vi "Capture System Configuration.vi"() -> ()   [LabVIEW 2024]
uses:
  <vilib>/nisyscfg/nisyscfg.lvlib
  <resource>/objmgr/nisysapi.rc
  <vilib>/Plug-In SDKs/Clients/Metadata Store V1/Metadata Store Client.lvlibp
  <vilib>/Plug-In SDKs/Clients/Metadata/Hardware Item.ctl
  <vilib>/Plug-In SDKs/Clients/Metadata/NI Metadata Types.lvlib
  <vilib>/Plug-In SDKs/Clients/Metadata/Software Item.ctl
  <vilib>/Plug-In SDKs/Clients/Metadata/Test Station.ctl
  <vilib>/Plug-In SDKs/Clients/Data Store V1/Data Store Client.lvlibp
  <vilib>/Plug-In SDKs/Clients/Metadata/Outcome.ctl
  <vilib>/Plug-In SDKs/Clients/Data Store V1/Data Store Client.lvlibp/API/Data Store V1/Test Result.ctl
  <vilib>/Plug-In SDKs/Clients/Metadata/Operator.ctl
  State Data.ctl
  <vilib>/Plug-In SDKs/Clients/Metadata/Step.ctl
  <vilib>/measure/NI_MABase.lvlib
  <vilib>/Plug-In SDKs/Clients/Metadata/Error Information.ctl
  <vilib>/Plug-In SDKs/Clients/Metadata/Extension Value.ctl
  <vilib>/Plug-In SDKs/Clients/Data Store V1/Data Store Client.lvlibp/API/Data Store V1/Publish Measurement (DBL Analog Waveform).vi
  <vilib>/Plug-In SDKs/Clients/Metadata Store V1/Metadata Store Client.lvlibp/API/Metadata Store V1/Create Hardware Item.vi
  <vilib>/Plug-In SDKs/Clients/Metadata Store V1/Metadata Store Client.lvlibp/API/Metadata Store V1/Create Software Item.vi
  <vilib>/nisyscfg/Get Installed Components.vi
  <vilib>/Plug-In SDKs/Clients/Metadata Store V1/Metadata Store Client.lvlibp/API/Metadata Store V1/Create Test Station.vi
  <vilib>/Plug-In SDKs/Clients/Metadata Store V1/Metadata Store Client.lvlibp/API/Metadata Store V1/Create Operator.vi
  <vilib>/Plug-In SDKs/Clients/Data Store V1/Data Store Client.lvlibp/API/Data Store V1/Read Data from Measurement (DBL Analog Waveform).vi
  <vilib>/Plug-In SDKs/Clients/Metadata Store V1/Metadata Store Client.lvlibp/API/Metadata Store V1/Get Operator.vi
  <vilib>/Plug-In SDKs/Clients/Metadata Store V1/Metadata Store Client.lvlibp/API/Metadata Store V1/Get Test Station.vi
  <vilib>/Plug-In SDKs/Clients/Metadata Store V1/Metadata Store Client.lvlibp/API/Metadata Store V1/Get Software Item.vi
  <vilib>/Plug-In SDKs/Clients/Metadata Store V1/Metadata Store Client.lvlibp/API/Metadata Store V1/Get Hardware Item.vi
panel:
  out "found operator":T1
  out "found software items":T3[](array[typedef])
  out "found hardware items":T4[](array[typedef])
  out "found test station":T5
  out "queried data":waveform(dbl)(graph)
  out "error out":errorcluster
  # "Capture System Configuration\n\nThis example uses System API to query information about the current system and create metadata items based on that information. A waveform measurement is published, then the data and metadata are read back from the published measurement."
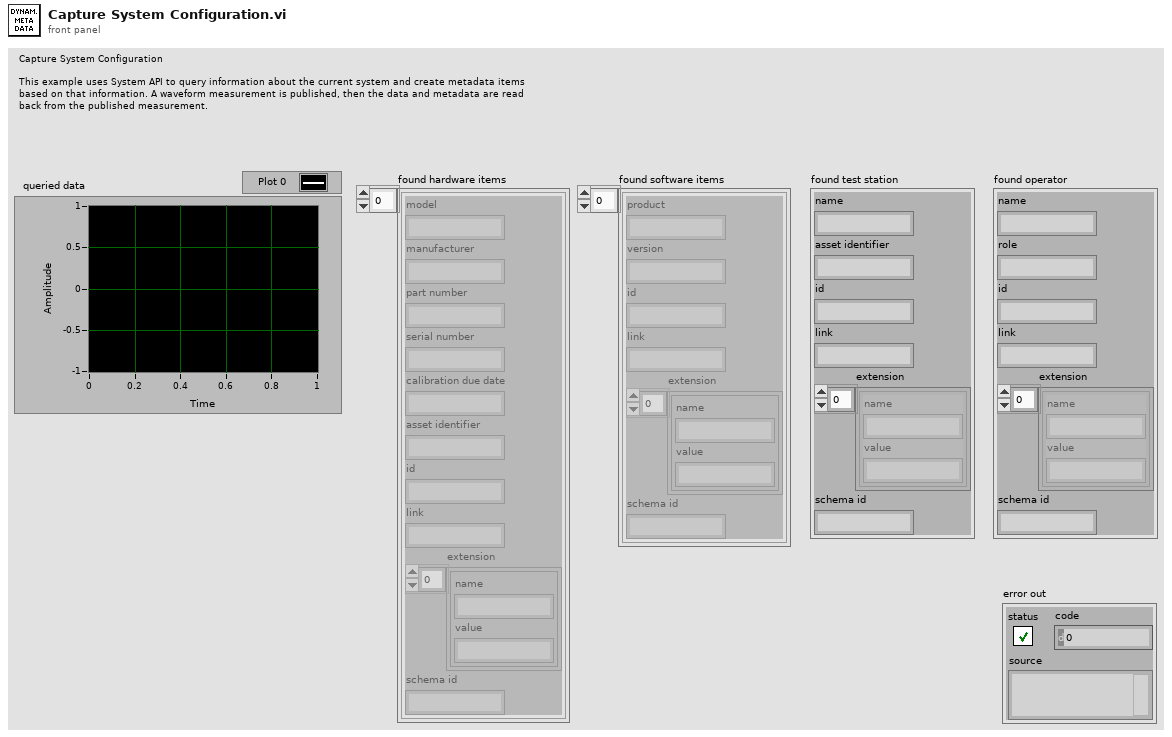
[diagram p1: front panel]
types:
  T1 = typedef "NI Metadata Types.lvlib/Operator.ctl" = cluster{"name":string, "role":string, "id":string, "link":string, "extension":T2[], "schema id":string}
  T2 = typedef "NI Metadata Types.lvlib/Extension Value.ctl" = cluster{"name":string, "value":string}
  T3 = typedef "NI Metadata Types.lvlib/Software Item.ctl" = cluster{"product":string, "version":string, "id":string, "link":string, "extension":T2[], "schema id":string}
  T4 = typedef "NI Metadata Types.lvlib/Hardware Item.ctl" = cluster{"model":string, "manufacturer":string, "part number":string, "serial number":string, "calibration due date":string, "asset identifier":string, "id":string, "link":string, "extension":T2[], "schema id":string}
  T5 = typedef "NI Metadata Types.lvlib/Test Station.ctl" = cluster{"name":string, "asset identifier":string, "id":string, "link":string, "extension":T2[], "schema id":string}
  T6 = typedef "State Data.ctl" = cluster{"operator id":string, "test station id":string, "hardware item ids":string[], "software item ids":string[], "test result id":string}
  T7 = enum16{"Find Hardware Items", "Find Software Items", "Find Test Station", "Find Operator", "Create Test Result", "Publish and Read Measurement", "Query Metadata"}
  T8 = typedef "Environment Values.ctl" = cluster{"cluster id":string, "failed ingest dir":string, "data files dir":string, "ingest dir":string, "db path":string, "cache expiration":string}
  T9 = typedef "Data Store Client.lvlibp/Test Result.ctl" = cluster{"name":string, "start date time":timestamp, "end date time":timestamp, "outcome":T10, "error information":T11, "id":string, "uut instance id":string, "operator id":string, "test station id":string, "test description id":string, "software item ids":string[], "hardware item ids":string[], "test adapter ids":string[], "link":string, "extension":T2[], "schema id":string}
  T10 = typedef "NI Metadata Types.lvlib/Outcome.ctl" = enum32{"Unspecified", "Passed", "Failed", "Indeterminate"}
  T11 = typedef "NI Metadata Types.lvlib/Error Information.ctl" = cluster{"error code":i32, "message":string, "source":string}
  T12 = typedef "NI Metadata Types.lvlib/Step.ctl" = cluster{"name":string, "step type":string, "start date time":timestamp, "end date time":timestamp, "notes":string, "outcome":T10, "error information":T11, "id":string, "parent step id":string, "test result id":string, "test id":string, "link":string, "extension":T2[], "schema id":string}
  T13 = typedef "nisyscfg.lvlib/Software 1.2.ctl" = cluster{"title":string, "description":string, "ID":string, "version":string, "component type":T14}
  T14 = typedef "nisyscfg.lvlib/Component Type.ctl" = u32
  T15 = typedef "Data Store Client.lvlibp/Published Measurement.ctl" = cluster{"parametric index":i32, "name":string, "value type":string, "notes":string, "start date time":timestamp, "end date time":timestamp, "outcome":T10, "error information":T11, "published conditions":T16[], "data moniker":T17, "id":string, "test result id":string, "step id":string, "software item ids":string[], "hardware item ids":string[], "test adapter ids":string[]}
  T16 = typedef "Data Store Client.lvlibp/Published Condition.ctl" = cluster{"name":string, "condition type":string, "moniker":T17, "id":string, "step id":string, "test result id":string}
  T17 = typedef "Data Store Client.lvlibp/Data Moniker.ctl" = cluster{"service location":string, "data source":string, "data instance":i64}
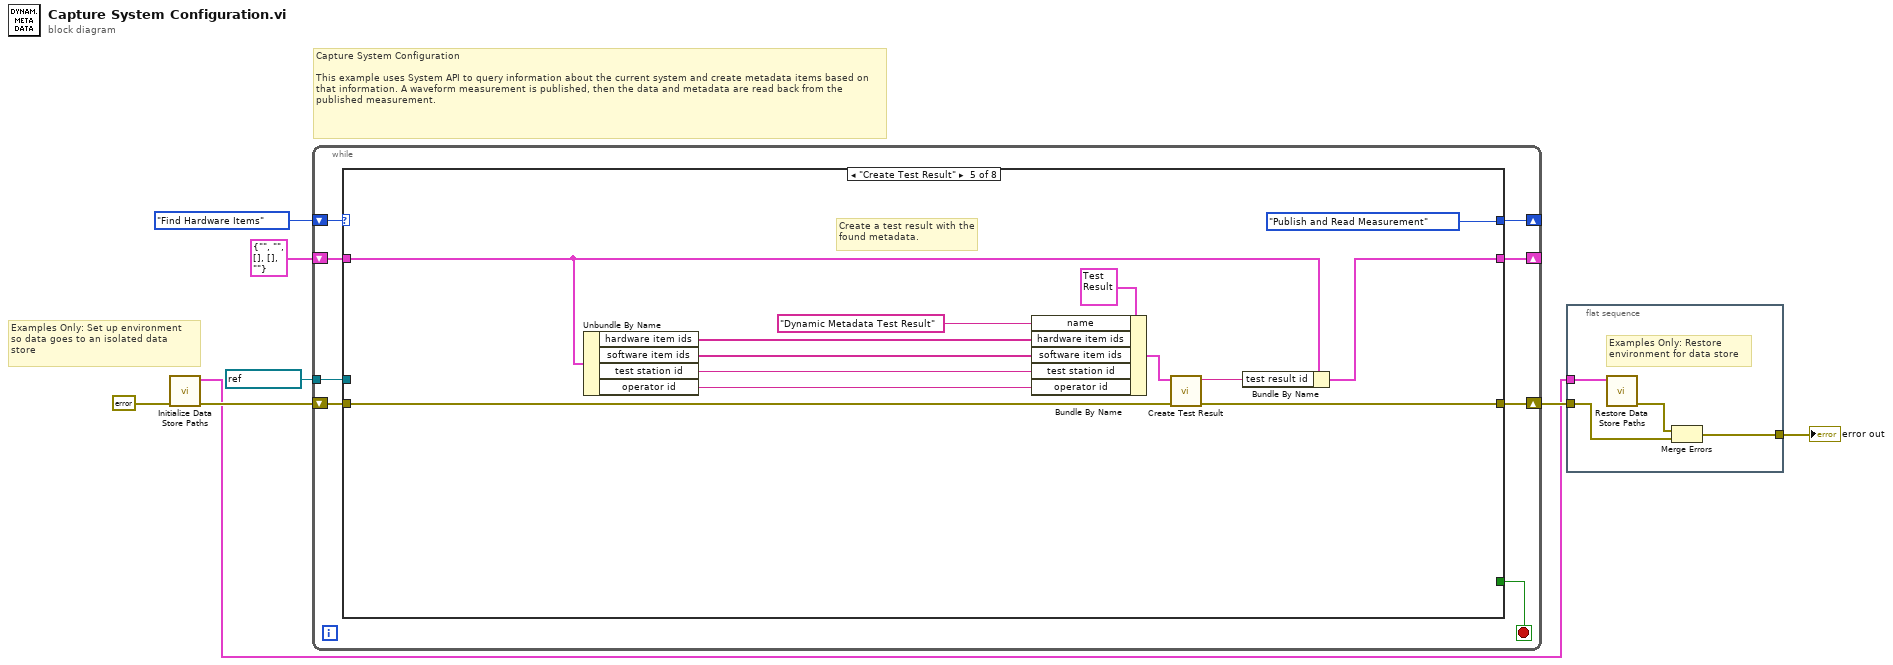
[diagram p0: block diagram]
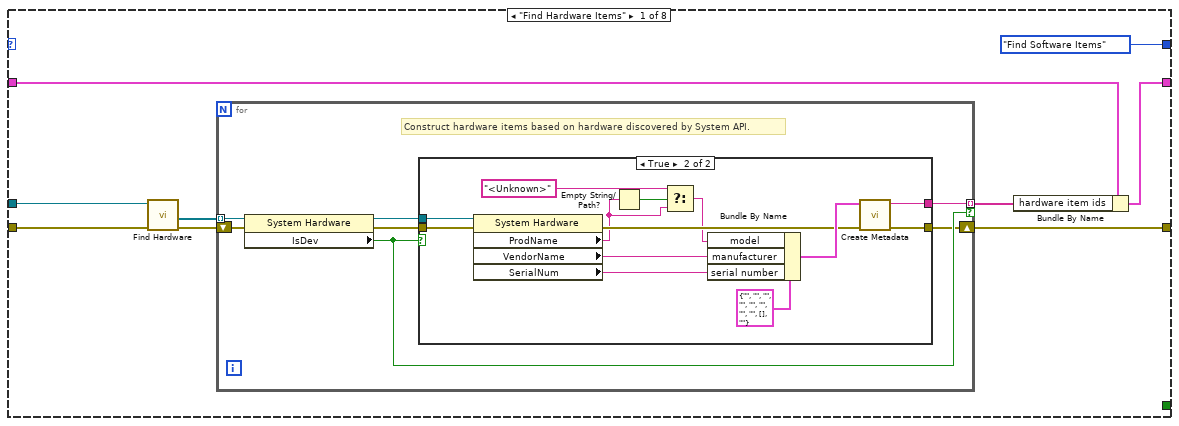
[diagram p2: hidden frame]
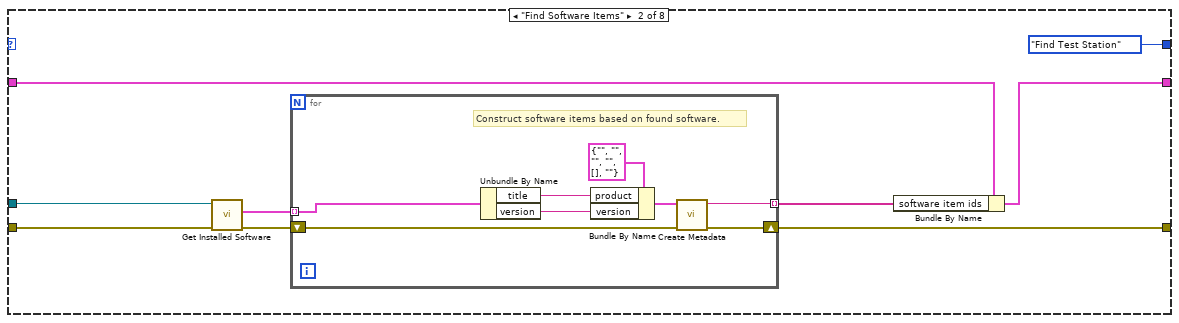
[diagram p4: hidden frame]
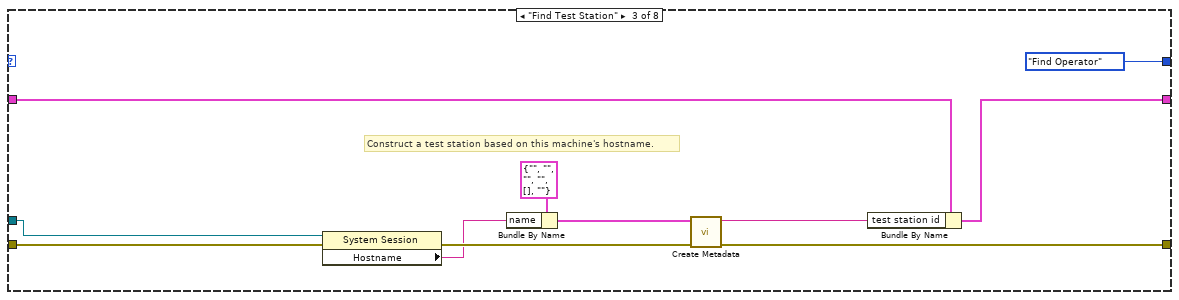
[diagram p5: hidden frame]
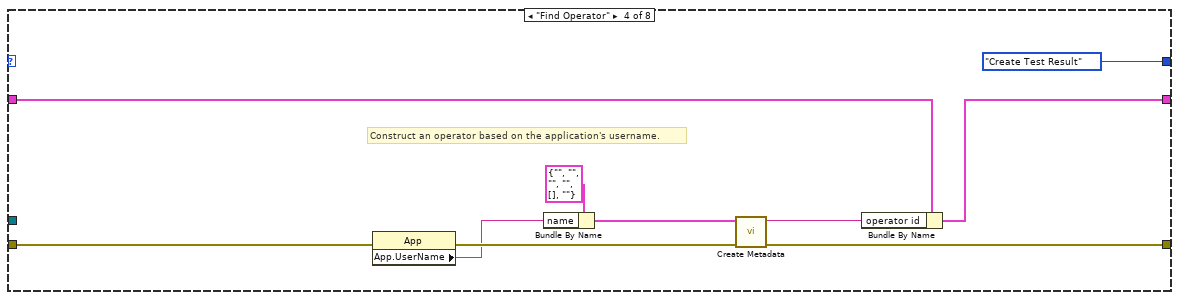
[diagram p6: hidden frame]
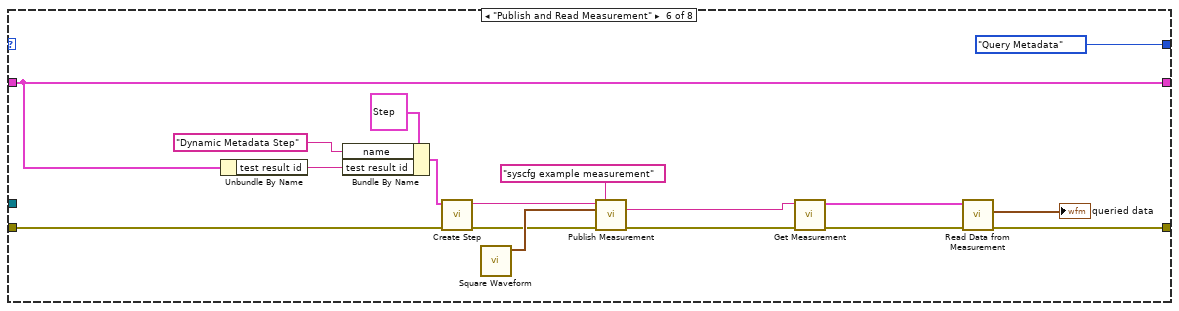
[diagram p7: hidden frame]
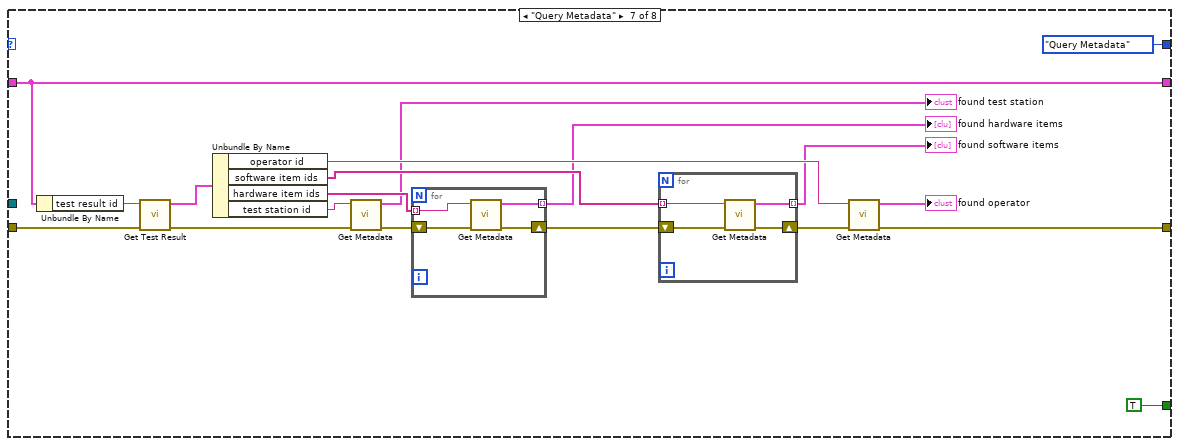
[diagram p8: hidden frame]
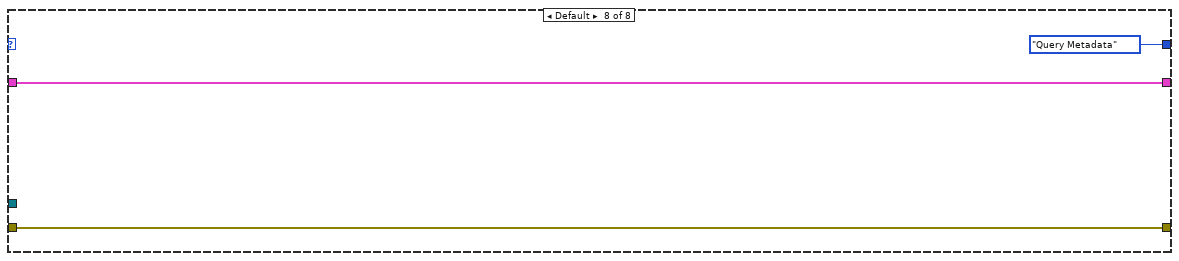
[diagram p9: hidden frame]
diagram:
  # "Examples Only: Set up environment\nso data goes to an isolated data\nstore"
  # "Capture System Configuration\n\nThis example uses System API to query information about the current system and create metadata items based on that information. A waveform measurement is published, then the data and metadata are read back from the published measurement."
  n1 = call "Initialize Data Store Paths.vi"("error in"=errorcluster {"status"=FALSE, "code"=0, "source"=""} ("error out")) -> ("error out"=w4:errorcluster, "original values"=w1:T8)  [unwired: 9 in]
  n2 = while {
    shift-right: [w13] -> _
    shift-left: T7."Find Hardware Items" -> [w14]
    shift-right: [w16] -> w3
    shift-left: w4 -> [w15]
    shift-right: [w11] -> _
    shift-left: T6 {"operator id"="", "test station id"="", "hardware item ids"=[], "software item ids"=[], "test result id"=""} ("State Data") -> [w12]
    tunnel: refnum<k21> "localhost" ("Session in") -> [w10]
    stop <- w9 stop-if-true
    n3 = case shown="\"Create Test Result\"" w14 {
      tunnel: [w23 w52 w69 w79 w89 w105 w126 w142] -> w16
      tunnel: w15 -> [w22 w53 w70 w80 w85 w108 w119 w142]
      tunnel: [T7."Find Software Items" T7."Find Test Station" T7."Find Operator" T7."Create Test Result" T7."Publish and Read Measurement" T7."Query Metadata" T7."Query Metadata" T7."Query Metadata"] -> w13
      tunnel: w12 -> [w21 w50 w68 w78 w86 w103 w116 w143]
      tunnel: [w19 w49 w66 w76 w88 w103 w116 w143] -> w11
      tunnel: w10 -> [w18 w51 w64 _ _ _ _ _]
      tunnel: [_ _ _ _ _ _ TRUE _] -> w9
      frame "Find Hardware Items" {
        n4 = call <vilib>:"Find Hardware.vi"("error in (no error)"=w22, "Session in"=w18) -> ("error out"=w24:errorcluster, "Resources out"=w25:refnum<k20>[])  [unwired: 6 in, 2 out]
        n5 = for {
          tunnel: w25 -> [w32] mode=indexing
          tunnel: [w29] -> w20 mode=indexing if=w27
          shift-right: [w26] -> w23
          shift-left: w24 -> [w28]
          # "Construct hardware items based on hardware discovered by System API."
          n6 = property class="System Hardware"(reference=w32, error in=w28) -> (reference out=w30:refnum<k20>, error out=w31:errorcluster, "IsDev"=w27:bool)
          n7 = case shown="True" w27 {
            tunnel: w31 -> [w33 w46]
            tunnel: w30 -> [_ w45]
            tunnel: [_ w40] -> w29
            tunnel: [w33 w38] -> w26
            frame False {
            }
            frame True {
              n8 = property class="System Hardware"(reference=w45, error in=w46) -> (error out=w39:errorcluster, "ProdName"=w35:string, "VendorName"=w42:string, "SerialNum"=w41:string)  [unwired: 1 out]
              n9 = Empty String/Path?(string/path=w35) -> (empty?=w37:bool)
              n10 = Select(t="<Unknown>", s=w37, f=w35) -> (s? t:f=w36:string)
              n11 = Bundle By Name(cluster=T4 {"model"="", "manufacturer"="", "part number"="", "serial number"="", "calibration due date"="", "asset identifier"="", "id"="", "link"="", "extension"=[], "schema id"=""} ("hardware item"), "model"=w36, "manufacturer"=w42, "serial number"=w41) -> (w44:T4)
              n12 = call-poly <vilib>:"Create Metadata.vi"("error in"=w39, "hardware item"=w44) -> ("error out"=w38:errorcluster, "hardware item id"=w40:string)  [unwired: 8 in]
            }
          }
        }
        n13 = Bundle By Name(cluster=w21, "hardware item ids"=w20) -> (w19:T6)
      }
      frame "Find Software Items" {
        n14 = call-poly <vilib>:"Get Installed Software.vi"("error in (no error)"=w53, "Session in"=w51) -> ("error out"=w54:errorcluster, "Software Components"=w55:T13[])  [unwired: 7 in, 1 out]
        n15 = for {
          tunnel: w55 -> [w63] mode=indexing
          shift-right: [w57] -> w52
          shift-left: w54 -> [w58]
          tunnel: [w56] -> w48 mode=indexing
          # "Construct software items based on found software."
          n16 = Unbundle By Name(w63) -> ("title"=w61:string, "version"=w60:string)
          n17 = Bundle By Name(cluster=T3 {"product"="", "version"="", "id"="", "link"="", "extension"=[], "schema id"=""} ("software item"), "product"=w61, "version"=w60) -> (w59:T3)
          n18 = call-poly <vilib>:"Create Metadata.vi"("error in"=w58, "software item"=w59) -> ("error out"=w57:errorcluster, "software item id"=w56:string)  [unwired: 8 in]
        }
        n19 = Bundle By Name(cluster=w50, "software item ids"=w48) -> (w49:T6)
      }
      frame "Find Test Station" {
        # "Construct a test station based on this machine's hostname."
        n20 = property class="System Session"(reference=w64, error in=w70) -> (error out=w72:errorcluster, "Hostname"=w71:string)  [unwired: 1 out]
        n21 = Bundle By Name(cluster=T5 {"name"="", "asset identifier"="", "id"="", "link"="", "extension"=[], "schema id"=""} ("test station"), "name"=w71) -> (w73:T5)
        n22 = call-poly <vilib>:"Create Metadata.vi"("error in"=w72, "test station"=w73) -> ("error out"=w69:errorcluster, "test station id"=w67:string)  [unwired: 8 in]
        n23 = Bundle By Name(cluster=w68, "test station id"=w67) -> (w66:T6)
      }
      frame "Find Operator" {
        # "Construct an operator based on the application's username."
        n24 = property class="App"(error in=w80) -> (error out=w83:errorcluster, "App.UserName"=w81:string)  [unwired: 1 in, 1 out]
        n25 = Bundle By Name(cluster=T1 {"name"="", "role"="", "id"="", "link"="", "extension"=[], "schema id"=""} ("operator metadata"), "name"=w81) -> (w82:T1)
        n26 = call-poly <vilib>:"Create Metadata.vi"("error in"=w83, "operator metadata"=w82) -> ("error out"=w79:errorcluster, "operator id"=w77:string)  [unwired: 8 in]
        n27 = Bundle By Name(cluster=w78, "operator id"=w77) -> (w76:T6)
      }
      frame "Create Test Result" {
        # "Create a test result with the found metadata."
        n28 = Unbundle By Name(w86) -> ("hardware item ids"=w94:string[], "software item ids"=w93:string[], "test station id"=w92:string, "operator id"=w91:string)
        n29 = Bundle By Name(cluster=T9 {"name"="", "start date time"=timestamp(0 s since 1904-01-01), "end date time"=timestamp(0 s since 1904-01-01), "outcome"=enum."Unspecified", "error information"={"error code"=0, "message"="", "source"=""}, "id"="", "uut instance id"="", "operator id"="", "test station id"="", "test description id"="", "software item ids"=[], "hardware item ids"=[], "test adapter ids"=[], "link"="", "extension"=[], "schema id"=""} ("test result"), "name"="Dynamic Metadata Test Result" ("test result name"), "hardware item ids"=w94, "software item ids"=w93, "test station id"=w92, "operator id"=w91) -> (w95:T9)
        n30 = call <vilib>:"Create Test Result.vi"("error in"=w85, "test result"=w95) -> ("error out"=w89:errorcluster, "test result id"=w90:string)  [unwired: 8 in]
        n31 = Bundle By Name(cluster=w86, "test result id"=w90) -> (w88:T6)
      }
      frame "Publish and Read Measurement" {
        n32 = Unbundle By Name(w103) -> ("test result id"=w107:string)
        n33 = Bundle By Name(cluster=T12 {"name"="", "step type"="", "start date time"=timestamp(0 s since 1904-01-01), "end date time"=timestamp(0 s since 1904-01-01), "notes"="", "outcome"=enum."Unspecified", "error information"={"error code"=0, "message"="", "source"=""}, "id"="", "parent step id"="", "test result id"="", "test id"="", "link"="", "extension"=[], "schema id"=""} ("step"), "name"="Dynamic Metadata Step" ("step name"), "test result id"=w107) -> (w111:T12)
        n34 = call <vilib>:"Create Step.vi"("error in"=w108, "step"=w111) -> ("error out"=w112:errorcluster, "step id"=w113:string)  [unwired: 8 in]
        n35 = call <vilib>:"Square Waveform.vi"() -> ("signal out"=w114:waveform(dbl))  [unwired: 10 in, 1 out]
        n36 = call-poly <vilib>:"Publish Measurement.vi"("step id"=w113, "name"="syscfg example measurement", "waveform"=w114, "error in"=w112) -> ("measurement id"=w99:string, "error out"=w101:errorcluster)  [unwired: 9 in, 1 out]
        n37 = call <vilib>:"Get Measurement.vi"("error in"=w101, "measurement id"=w99) -> ("error out"=w100:errorcluster, "published measurement"=w98:T15)  [unwired: 8 in]
        n38 = call-poly <vilib>:"Read Data from Measurement.vi"("error in"=w100, "published measurement"=w98) -> ("error out"=w105:errorcluster, "waveform data"=→"queried data":waveform(dbl))  [unwired: 7 in, 1 out]
      }
      frame "Query Metadata" {
        n39 = Unbundle By Name(w116) -> ("test result id"=w115:string)
        n40 = call <vilib>:"Get Test Result.vi"("error in"=w119, "test result id"=w115) -> ("error out"=w118:errorcluster, "test result"=w117:T9)  [unwired: 8 in]
        n41 = Unbundle By Name(w117) -> ("operator id"=w127:string, "software item ids"=w133:string[], "hardware item ids"=w131:string[], "test station id"=w129:string)
        n42 = call-poly <vilib>:"Get Metadata.vi"("error in"=w118, "test station id"=w129) -> ("error out"=w130:errorcluster, "test station metadata"=→"found test station":T5)  [unwired: 8 in]
        n43 = for {
          shift-right: [w140] -> w132
          shift-left: w130 -> [w141]
          tunnel: w131 -> [w139] mode=indexing
          tunnel: [w138] -> w124 mode=indexing
          n44 = call-poly <vilib>:"Get Metadata.vi"("error in"=w141, "hardware item id"=w139) -> ("error out"=w140:errorcluster, "hardware item"=w138:T4)  [unwired: 8 in]
        }
        "found hardware items" <- w124
        n45 = for {
          shift-right: [w136] -> w128
          shift-left: w132 -> [w137]
          tunnel: w133 -> [w135] mode=indexing
          tunnel: [w134] -> w123 mode=indexing
          n46 = call-poly <vilib>:"Get Metadata.vi"("error in"=w137, "software item id"=w135) -> ("error out"=w136:errorcluster, "software item"=w134:T3)  [unwired: 8 in]
        }
        "found software items" <- w123
        n47 = call-poly <vilib>:"Get Metadata.vi"("error in"=w128, "operator id"=w127) -> ("error out"=w126:errorcluster, "operator metadata"=→"found operator":T1)  [unwired: 8 in]
      }
      frame Default {
      }
    }
  }
  n48 = flat-sequence {
    tunnel: w1 -> [w148]
    tunnel: w3 -> [w146]
    tunnel: [w145] -> w2
    frame #0 {
      # "Examples Only: Restore\nenvironment for data store"
      n49 = call "Restore Data Store Paths.vi"("original values"=w148) -> ("error out"=w147:errorcluster)  [unwired: 10 in]
      n50 = Merge Errors(w147, w146) -> (w145:errorcluster)
    }
  }
  "error out" <- w2
